vi "test_grab_video.vi"() -> ()   [LabVIEW 2015]
panel:
  in  "Boolean":bool
  in  "stop":bool
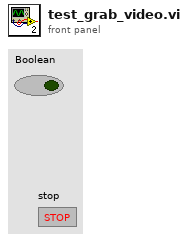
[diagram p1: front panel]
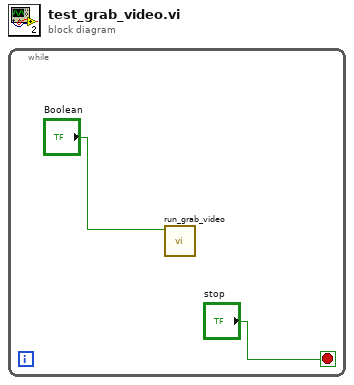
[diagram p0: block diagram]
diagram:
  n1 = while {
    stop <- "stop" stop-if-true
    n2 = call "run_grab_video.vi"("Input"="Boolean") -> ()  [unwired: 11 in]
  }
